vi "Actuateur.vi"(1 "Actuateur Arrière":bool, 2 "Actuateur Avant":bool) -> ()   [LabVIEW 2018]
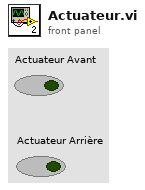
[diagram p1: front panel]
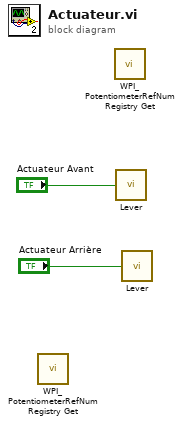
[diagram p0: block diagram]
diagram:
  n1 = call <vilib>:"WPI_PotentiometerRefNum Registry Get.vi"() -> ()  [unwired: 10 in, 2 out]
  n2 = call <vilib>:"WPI_PotentiometerRefNum Registry Get.vi"() -> ()  [unwired: 10 in, 2 out]
  n3 = call "Lever.vi"("Input"="Actuateur Avant") -> ()  [unwired: 1 out]
  n4 = call "Lever.vi"("Input"="Actuateur Arrière") -> ()  [unwired: 1 out]
